vi "Open Block Diagram.vi"(8 "error in (no error)":errorcluster, 9 "Assertion Label":string, 10 "Call Chain":string[](array[string]), 11 "Basic Test Manager in":refnum<class "Basic Test Manager.lvclass">) -> (0 "error out":errorcluster, 3 "Basic Test Manager out":refnum<class "Basic Test Manager.lvclass">)   [LabVIEW 2013, in "Caraya.lvlib" / "Basic Test Manager.lvclass"]
uses:
  Basic Test Manager.lvclass
  <vilib>/regexp/Match Regular Expression.xnode
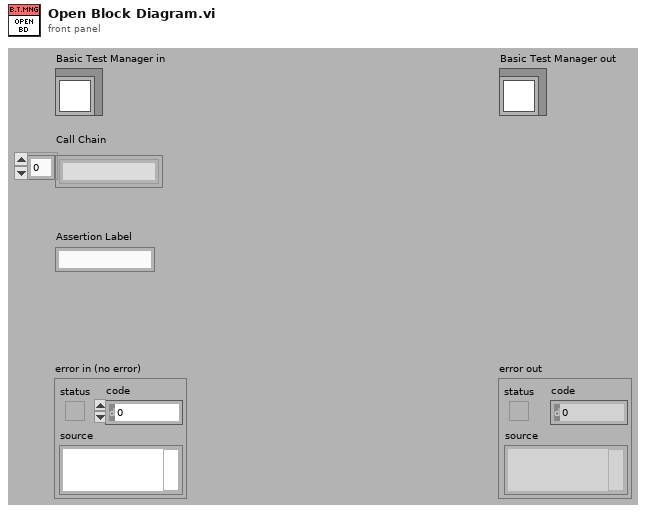
[diagram p1: front panel]
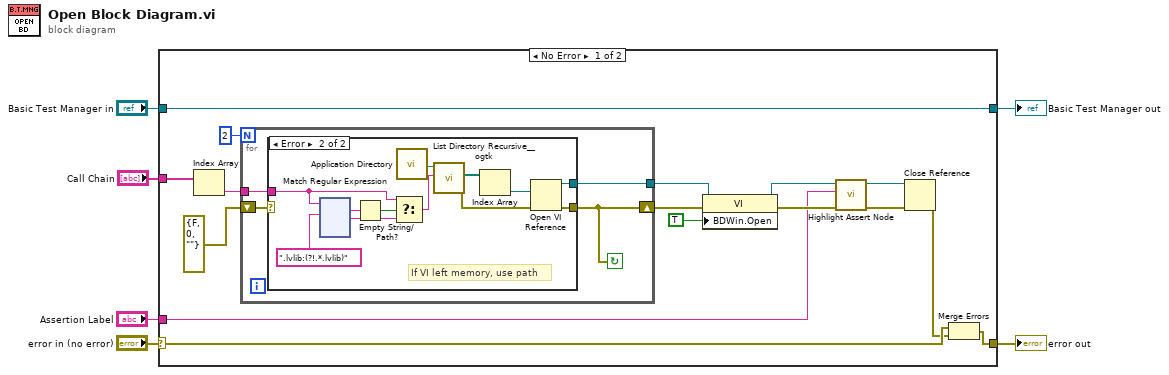
[diagram p0: block diagram]
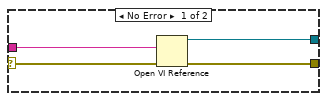
[diagram p2: hidden frame]
diagram:
  n1 = case shown="No Error" "error in (no error)" {
    selector: "error in (no error)" -> [w16 w158]
    tunnel: [w14 w158] -> w5
    tunnel: [w22 w157] -> w3
    tunnel: "Basic Test Manager in" -> [w22 w157]
    tunnel: "Call Chain" -> [w8 _]
    tunnel: "Assertion Label" -> [w9 _]
    frame No Error {
      n2 = Index Array(array=w8) -> (element=w7:string)  [unwired: 1 in]
      n3 = for {
        N: 2 -> [_]
        tunnel: [w26] -> w21
        tunnel: w7 -> [w25]
        shift-right: [w24] -> w20
        shift-left: errorcluster {"status"=FALSE, "code"=0, "source"=""} ("error out") -> [w23]
        stop <- w24 continue-if-true
        n4 = case shown="Error" w23 {
          selector: w23 -> [w27 _]
          tunnel: [w30 w41] -> w26
          tunnel: w25 -> [w29 w32]
          tunnel: [w28 w42] -> w24
          frame No Error {
            n5 = Open VI Reference(vi path=w29, error in (no error)=w27) -> (vi reference=w30:refnum<vi>, error out=w28:errorcluster)  [unwired: 4 in]
          }
          frame Error {
            # "If VI left memory, use path"
            n6 = xnode "Match Regular Expression"("input string"=w32, "regular expression"=".lvlib:(?!.*.lvlib)") -> ("whole match"=w34:string, "after match"=w33:string)  [unwired: 4 in, 3 out]
            n7 = Empty String/Path?(string/path=w34) -> (empty?=w36:bool)
            n8 = Select(t=w32, s=w36, f=w33) -> (s? t:f=w35:string)
            n9 = call <vilib>:"Application Directory.vi"() -> ("Application Directory"=w37:path)
            n10 = call <userlib>:"List Directory Recursive__ogtk.vi"("pattern"=w35, "Path"=w37) -> ("error out"=w38:errorcluster, "file paths"=w40:path[])  [unwired: 6 in, 2 out]
            n11 = Index Array(array=w40) -> (element=w39:path)  [unwired: 1 in]
            n12 = Open VI Reference(vi path=w39, error in (no error)=w38) -> (vi reference=w41:refnum<vi>, error out=w42:errorcluster)  [unwired: 4 in]
          }
        }
      }
      n13 = property class="VI"(reference=w21, error in=w20, "BDWin.Open"=TRUE ("Block Diagram Window:Open")) -> (reference out=w13:refnum<vi>, error out=w11:errorcluster)
      n14 = call "Highlight Assert Node.vi"("error in (no error)"=w11, "Assertion Label"=w9, "vi reference"=w13) -> ("error out"=w10:errorcluster, "vi reference  dup"=w12:refnum<vi>)  [unwired: 7 in]
      n15 = Close Reference(reference=w12, error in (no error)=w10) -> (error out=w15:errorcluster)
      n16 = Merge Errors(w16, w15) -> (w14:errorcluster)
    }
    frame Error {
    }
  }
  "error out" <- w5
  "Basic Test Manager out" <- w3
